vi "Tank Drive Reduce Speed Button.vi"(7 "Reduce By (Default 2)":dbl=2.0, 8 "R-In":dbl(slide) scale=-1.0..1.0, 10 "Reduce Speed":bool, 11 "L- In":dbl(slide) scale=-1.0..1.0) -> (0 "R-out":dbl(slide) scale=-1.0..1.0, 3 "L-Out":dbl(slide) scale=-1.0..1.0)   [LabVIEW 2011]
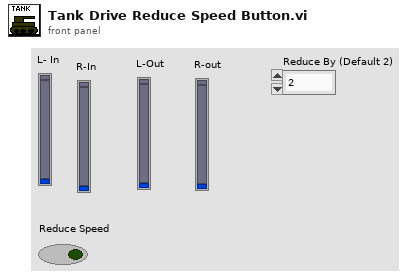
[diagram p1: front panel]
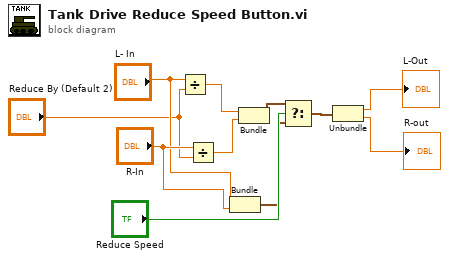
[diagram p0: block diagram]
diagram:
  n1 = Divide(x="L- In", y="Reduce By (Default 2)") -> (x/y=w6:dbl)
  n2 = Divide(x="R-In", y="Reduce By (Default 2)") -> (x/y=w5:dbl)
  n3 = Bundle("L- In"="L- In", "R-In"="R-In") -> (w4:cluster{"L- In":dbl, "R-In":dbl})  [unwired: 1 in]
  n4 = Bundle(w6, w5) -> (w7:cluster{dbl, dbl})  [unwired: 1 in]
  n5 = Select(t=w7, s="Reduce Speed", f=w4) -> (s? t:f=w10:cluster{"L- In":dbl, "R-In":dbl})
  n6 = Unbundle(w10) -> ("L- In"=→"L-Out":dbl, "R-In"=→"R-out":dbl)
